vi "Configure Instrument.vi"(8 "error in (no error)":errorcluster, 11 "Example Instrument in":refnum<class "ExampleInstrument.lvclass">) -> (0 "error out":errorcluster, 3 "Example Instrument out":refnum<class "ExampleInstrument.lvclass">)   [LabVIEW 2016, in "ExampleInstrument.lvclass"]
uses:
  ExampleInstrument.lvclass
  ExampleInstrument.lvclass/ExampleInstrument.ctl
  lvsrc/SMOs/Instrument/Instrument.lvclass
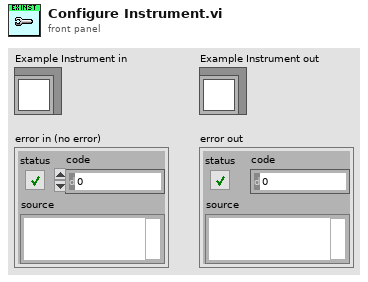
[diagram p1: front panel]
types:
  T1 = typedef "ExampleInstrument.lvclass/ExampleInstrument.Configuration--Cluster.ctl" = cluster{"Example Setting 1":dbl, "Example Setting 2":dbl, "Example Setting 3":string}
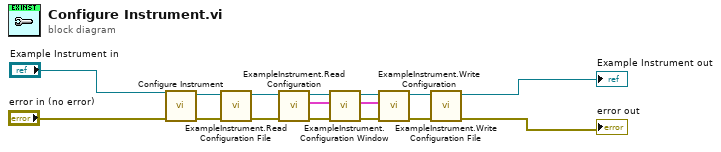
[diagram p0: block diagram]
diagram:
  n1 = call-parent "Configure Instrument.vi"("error in (no error)"="error in (no error)", "Instrument in"="Example Instrument in") -> ("error out"=w11:errorcluster, "Instrument out"=w13:refnum<class "ExampleInstrument.lvclass">)  [unwired: 8 in]
  n2 = call "ExampleInstrument.Read Configuration File.vi"("error in (no error)"=w11, "Example Instrument in"=w13) -> ("error out"=w10:errorcluster, "Example Instrument out"=w9:refnum<class "ExampleInstrument.lvclass">)  [unwired: 8 in]
  n3 = call "ExampleInstrument.Read Configuration.vi"("error in (no error)"=w10, "Example Instrument in"=w9) -> ("error out"=w7:errorcluster, "Configuration"=w2:T1, "Example Instrument out"=w8:refnum<class "ExampleInstrument.lvclass">)  [unwired: 7 in]
  n4 = call "ExampleInstrument.Configuration Window.vi"("error in (no error)"=w7, "Ex Configuration"=w2, "Example Instrument in"=w8) -> ("error out"=w6:errorcluster, "output cluster"=w1:T1, "Example Instrument out"=w5:refnum<class "ExampleInstrument.lvclass">)  [unwired: 6 in]
  n5 = call "ExampleInstrument.Write Configuration.vi"("error in (no error)"=w6, "Configuration"=w1, "Example Instrument in"=w5) -> ("error out"=w3:errorcluster, "Example Instrument out"=w4:refnum<class "ExampleInstrument.lvclass">)  [unwired: 7 in]
  n6 = call "ExampleInstrument.Write Configuration File.vi"("error in (no error)"=w3, "Example Instrument in"=w4) -> ("error out"=→"error out":errorcluster, "Example Instrument out"=→"Example Instrument out":refnum<class "ExampleInstrument.lvclass">)  [unwired: 8 in]
